vi "Process Collision.vi"(11 "Collision in":refnum<class "Collision.lvclass">) -> (3 "Collision out":refnum<class "Collision.lvclass">)   [LabVIEW 2021, in "Collision.lvclass"]
doc: "MIT Licence\nCopyright (c) 2024 David Grollier"
uses:
  Collision.lvclass
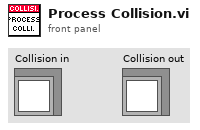
[diagram p1: front panel]
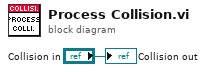
[diagram p0: block diagram]
diagram:
  "Collision out" <- "Collision in"
